vi "Compile Routines.vi"(8 "error in (no error)":errorcluster, 9 "Routines":T5[](array[typedef]) {"Stop Parameters"."Response"."Byte Order" items=["Little Endian", "Big Endian"]; "Stop Parameters"."Response"."Data Type" items=["Signed", "Unsigned", "IEEE Float"]; "Stop Parameters"."Cmd"."Byte Order" items=["Little Endian", "Big Endian"]; "Stop Parameters"."Cmd"."Data Type" items=["Signed", "Unsigned", "IEEE Float"]; "Request Parameters"."Response"."Byte Order" items=["Little Endian", "Big Endian"]; "Request Parameters"."Response"."Data Type" items=["Signed", "Unsigned", "IEEE Float"]; "Request Parameters"."Cmd"."Byte Order" items=["Little Endian", "Big Endian"]; "Request Parameters"."Cmd"."Data Type" items=["Signed", "Unsigned", "IEEE Float"]; "Start Parameters"."Response"."Byte Order" items=["Little Endian", "Big Endian"]; "Start Parameters"."Response"."Data Type" items=["Signed", "Unsigned", "IEEE Float"]; "Start Parameters"."Cmd"."Byte Order" items=["Little Endian", "Big Endian"]; "Start Parameters"."Cmd"."Data Type" items=["Signed", "Unsigned", "IEEE Float"]}, 10 "Routine Refs":T8[](array[typedef]) {"Stop"."Cmd Refs" format="%.0x"; "Stop"."Resp Refs" format="%.0x"; "Status"."Cmd Refs" format="%.0x"; "Status"."Resp Refs" format="%.0x"; "Start"."Cmd Refs" format="%.0x"; "Start"."Resp Refs" format="%.0x"}, 11 "Item Ref in":T10 format="%.0x") -> (0 "error out":errorcluster, 1 "Refs":T2 {"Stop.Resp" format="%.0x"; "Stop.Cmds"."Refs"."Data Reference" format="%.0x"; "Request.Resp" format="%.0x"; "Request.Cmds"."Refs"."Data Reference" format="%.0x"; "Start.Resp" format="%.0x"; "Start.Cmds"."Refs"."Data Reference" format="%.0x"}, 2 "Lookups":T1, 3 "Item Ref out":T10=18446744073709551615 format="%.0x")   [LabVIEW 2015, in "Diagnostics Addon System Explorer.lvlib"]
uses:
  Diagnostics Addon System Explorer.lvlib
  <vilib>/NI Veristand/Custom Device API/Custom Device Item Ref.ctl
  Types/Routine VS References.ctl
  Shared/Types/CmdResp Refs.ctl
  Shared/Types/Routine Paramaters.ctl
  Shared/Types/Command Response Signals.ctl
  Shared/Types/Signal Parameters.ctl
  Shared/Types/Compiled Routine Refs.ctl
  <vilib>/NI Veristand/Custom Device API/Block Data Reference.ctl
  <vilib>/NI Veristand/Custom Device API/Data Reference.ctl
  Shared/Types/Compiled Routine Lookups.ctl
  <vilib>/NI Veristand/Custom Device API/Data Access Type.ctl
  Shared/Types/Datatable Lookup Positions.ctl
  Shared/Diagnostics Addon Shared.lvlib
  <vilib>/NI Veristand/Custom Device API/Custom Device API.lvlib
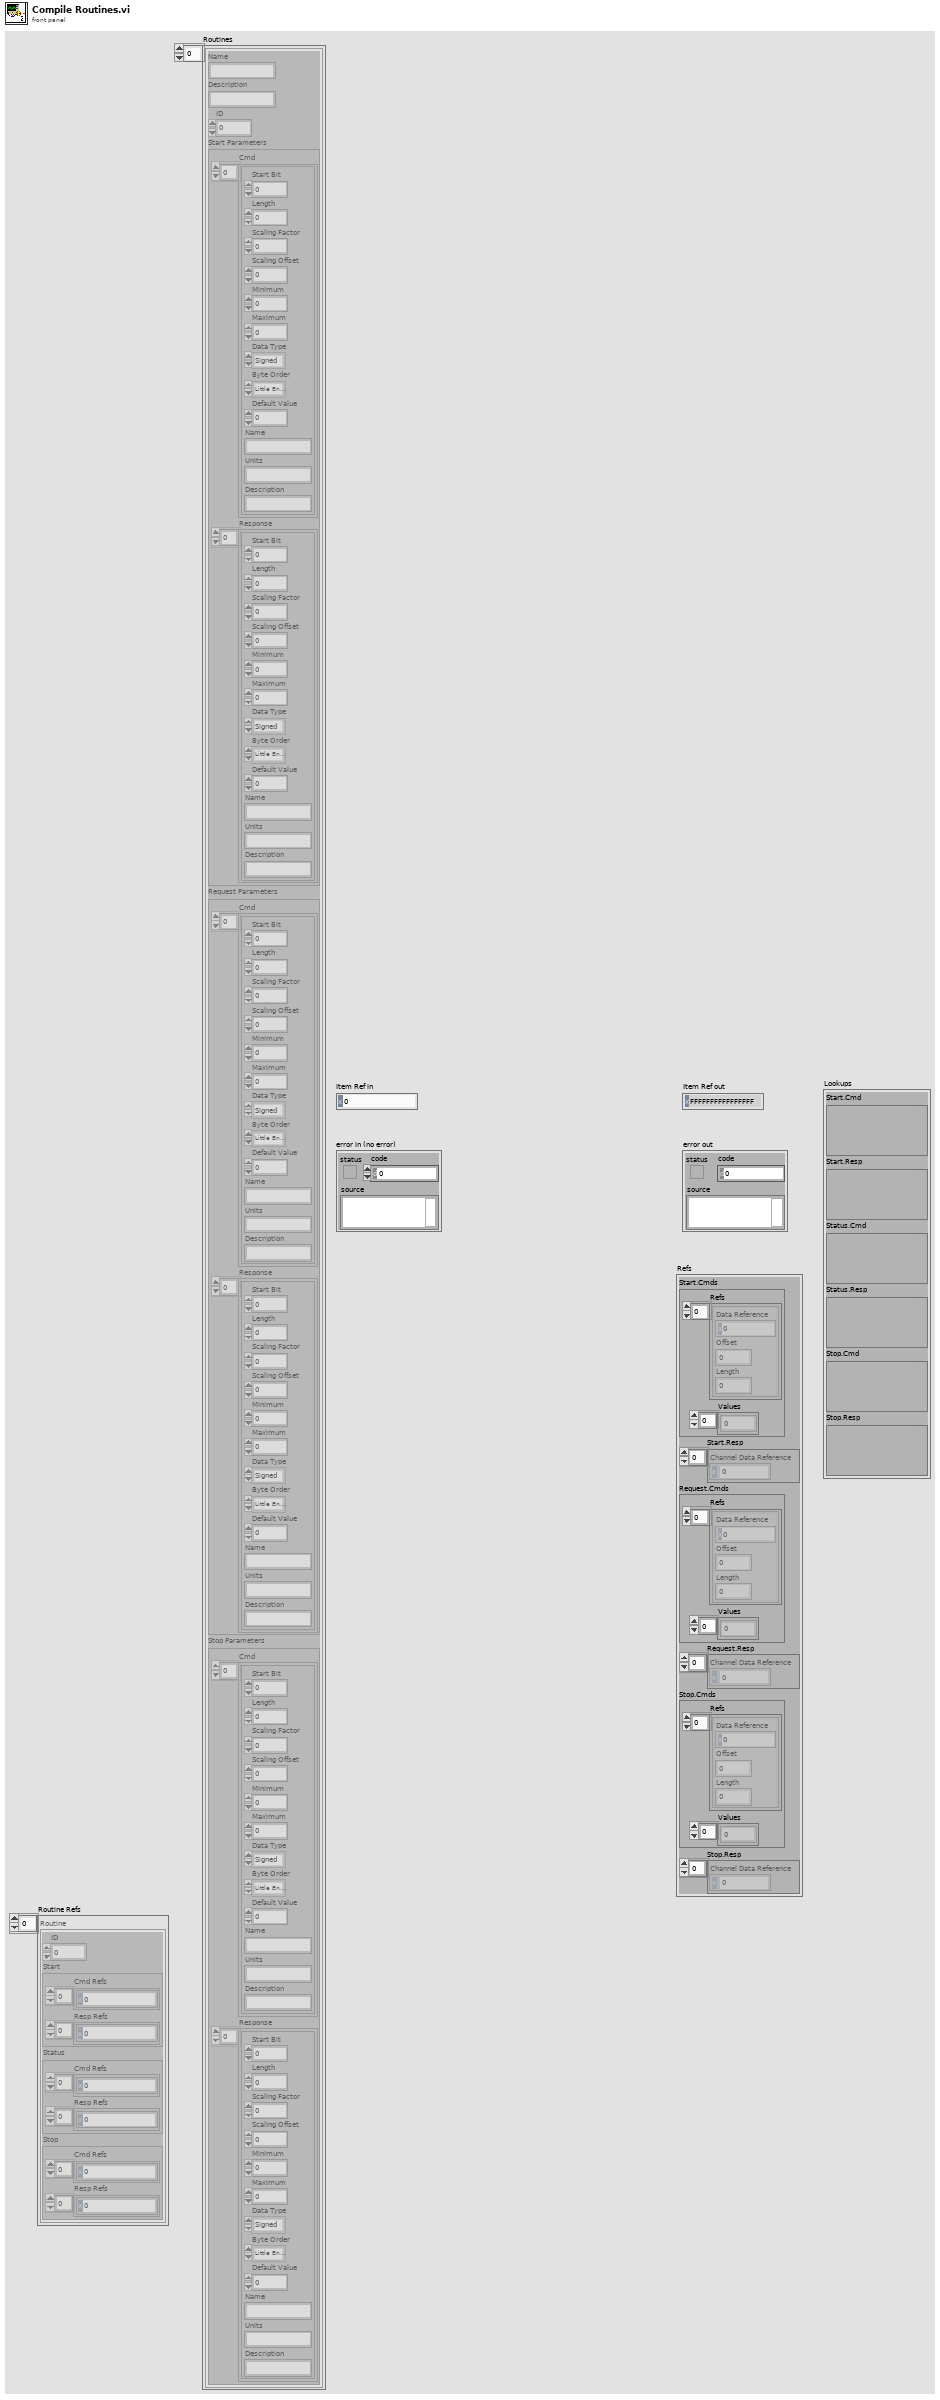
[diagram p1: front panel]
types:
  T1 = typedef "Diagnostics Addon Shared.lvlib/Compiled Routine Lookups.ctl" = cluster{"Start.Cmd":variant, "Start.Resp":variant, "Status.Cmd":variant, "Status.Resp":variant, "Stop.Cmd":variant, "Stop.Resp":variant}
  T2 = typedef "Diagnostics Addon Shared.lvlib/Compiled Routine Refs.ctl" = cluster{"Start.Cmds":cluster{"Refs":T3[], "Values":dbl[]}, "Start.Resp":T4[], "Request.Cmds":cluster{"Refs":T3[], "Values":dbl[]}, "Request.Resp":T4[], "Stop.Cmds":cluster{"Refs":T3[], "Values":dbl[]}, "Stop.Resp":T4[]}
  T3 = typedef "Custom Device API.lvlib/Block Data Reference.ctl" = cluster{"Data Reference":T4, "Offset":u64, "Length":u64}
  T4 = typedef "Custom Device API.lvlib/Data Reference.ctl" = i32
  T5 = typedef "Diagnostics Addon Shared.lvlib/Routine Paramaters.ctl" = cluster{"Name":string, "Description":string, "ID":u16, "Start Parameters":T6, "Request Parameters":T6, "Stop Parameters":T6}
  T6 = typedef "Diagnostics Addon Shared.lvlib/Command Response Signals.ctl" = cluster{"Cmd":T7[], "Response":T7[]}
  T7 = typedef "Diagnostics Addon Shared.lvlib/Signal Parameters.ctl" = cluster{"Start Bit":u8, "Length":u8, "Scaling Factor":dbl, "Scaling Offset":dbl, "Minimum":dbl, "Maximum":dbl, "Data Type":u32, "Byte Order":u32, "Default Value":dbl, "Name":string, "Units":string, "Description":string}
  T8 = typedef "Diagnostics Addon System Explorer.lvlib/Routine VS References.ctl" = cluster{"ID":u32, "Start":T9, "Status":T9, "Stop":T9}
  T9 = typedef "Diagnostics Addon Shared.lvlib/CmdResp Refs.ctl" = cluster{"Cmd Refs":T10[], "Resp Refs":T10[]}
  T10 = typedef "Custom Device API.lvlib/Custom Device Item Ref.ctl" = u64
  T11 = typedef "Custom Device API.lvlib/Data Access Type.ctl" = enum16{"Read", "Write"}
  T12 = typedef "Diagnostics Addon Shared.lvlib/Datatable Lookup Positions.ctl" = cluster{"Offset":i32, "Length":i32, "ByteLength":u16}
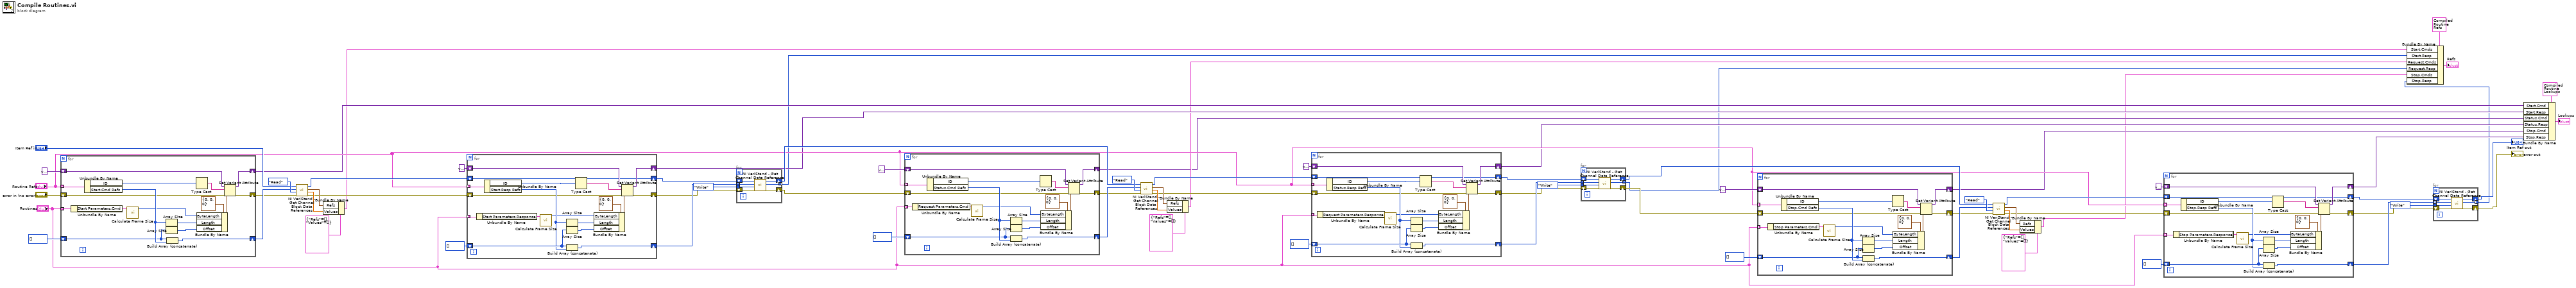
[diagram p0: block diagram]
diagram:
  n1 = for {
    tunnel: "Routine Refs" -> [w83] mode=indexing
    shift-right: [w84] -> w14
    shift-left: variant -> [w88]
    shift-right: [w86] -> w65
    shift-left: "error in (no error)" -> [w79]
    shift-right: [w82] -> w70
    shift-left: T10[] [] -> [w80]
    tunnel: "Routines" -> [w78] mode=indexing
    n2 = Unbundle By Name(w78) -> ("Start Parameters.Cmd"=w77:T7[])
    n3 = Unbundle By Name(w83) -> ("ID"=w75:u32, "Start.Cmd Refs"=w81:T10[])
    n4 = call "Calculate Frame Size.vi"("Parameters"=w77) -> ("Bytes"=w76:u16)  [unwired: 10 in]
    n5 = Array Size(array=w81) -> (size(s)=w91:i32)
    n6 = Array Size(array=w80) -> (size(s)=w87:i32)
    n7 = Build Array (concatenate)(w80, w81) -> (w82:T10[])
    n8 = Type Cast(x=w75) -> (*(type *) &x=w85:string)  [unwired: 1 in]
    n9 = Bundle By Name(cluster=T12 {"Offset"=0, "Length"=0, "ByteLength"=0}, "ByteLength"=w76, "Length"=w91, "Offset"=w87) -> (w89:T12)
    n10 = Set Variant Attribute(Variant=w88, name=w85, value=w89, error in=w79) -> (Variant out=w84:variant, error out=w86:errorcluster)  [unwired: 1 out]
  }
  n11 = call <vilib>:"NI VeriStand - Get Channel Block Data References.vi"("error in (no error)"=w65, "Access"=Data_Access_Type."Read", "Channel Refs"=w70, "Device Ref in"="Item Ref in") -> ("error out"=w58:errorcluster, "Values Array"=w66:dbl[], "Block Data Refs"=w67:T3[], "Device Ref out"=w57:T10)  [unwired: 4 in]
  n12 = Bundle By Name(cluster=cluster{"Refs":T3[], "Values":dbl[]} {"Refs"=[], "Values"=[]} ("Pairs"), "Refs"=w67, "Values"=w66) -> (w13:cluster{"Refs":T3[], "Values":dbl[]})
  n13 = for {
    tunnel: "Routine Refs" -> [w99] mode=indexing
    shift-right: [w108] -> w60
    shift-left: T10[] [] ("Signal Refs") -> [w109]
    shift-right: [w100] -> w12
    shift-left: variant -> [w104]
    shift-right: [w102] -> w59
    shift-left: w58 -> [w97]
    shift-right: [w96] -> w61
    shift-left: w57 -> [w96]
    tunnel: "Routines" -> [w95] mode=indexing
    n14 = Unbundle By Name(w95) -> ("Start Parameters.Response"=w94:T7[])
    n15 = Unbundle By Name(w99) -> ("ID"=w92:u32, "Start.Resp Refs"=w98:T10[])
    n16 = call "Calculate Frame Size.vi"("Parameters"=w94) -> ("Bytes"=w93:u16)  [unwired: 10 in]
    n17 = Array Size(array=w98) -> (size(s)=w107:i32)
    n18 = Array Size(array=w109) -> (size(s)=w103:i32)
    n19 = Build Array (concatenate)(w109, w98) -> (w108:T10[])
    n20 = Type Cast(x=w92) -> (*(type *) &x=w101:string)  [unwired: 1 in]
    n21 = Bundle By Name(cluster=T12 {"Offset"=0, "Length"=0, "ByteLength"=0}, "ByteLength"=w93, "Length"=w107, "Offset"=w103) -> (w105:T12)
    n22 = Set Variant Attribute(Variant=w104, name=w101, value=w105, error in=w97) -> (Variant out=w100:variant, error out=w102:errorcluster)  [unwired: 1 out]
  }
  n23 = for {
    tunnel: w60 -> [w112] mode=indexing
    tunnel: Data_Access_Type."Write" ("Access") -> [w111]
    shift-right: [w114] -> w26
    shift-left: w59 -> [w115]
    shift-right: [w116] -> w25
    shift-left: w61 -> [w113]
    tunnel: [w110] -> w11 mode=indexing
    n24 = call <vilib>:"NI VeriStand - Get Channel Data Reference.vi"("error in (no error)"=w115, "Access"=w111, "Channel Ref in"=w112, "Device Ref in"=w113) -> ("error out"=w114:errorcluster, "Channel Data Reference"=w110:T4, "Device Ref out"=w116:T10)  [unwired: 5 in]
  }
  n25 = for {
    tunnel: "Routine Refs" -> [w125] mode=indexing
    shift-right: [w126] -> w9
    shift-left: variant -> [w130]
    shift-right: [w128] -> w50
    shift-left: w26 -> [w121]
    shift-right: [w124] -> w54
    shift-left: T10[] [] -> [w122]
    tunnel: "Routines" -> [w120] mode=indexing
    n26 = Unbundle By Name(w120) -> ("Request Parameters.Cmd"=w119:T7[])
    n27 = Unbundle By Name(w125) -> ("ID"=w117:u32, "Status.Cmd Refs"=w123:T10[])
    n28 = call "Calculate Frame Size.vi"("Parameters"=w119) -> ("Bytes"=w118:u16)  [unwired: 10 in]
    n29 = Array Size(array=w123) -> (size(s)=w133:i32)
    n30 = Array Size(array=w122) -> (size(s)=w129:i32)
    n31 = Build Array (concatenate)(w122, w123) -> (w124:T10[])
    n32 = Type Cast(x=w117) -> (*(type *) &x=w127:string)  [unwired: 1 in]
    n33 = Bundle By Name(cluster=T12 {"Offset"=0, "Length"=0, "ByteLength"=0}, "ByteLength"=w118, "Length"=w133, "Offset"=w129) -> (w131:T12)
    n34 = Set Variant Attribute(Variant=w130, name=w127, value=w131, error in=w121) -> (Variant out=w126:variant, error out=w128:errorcluster)  [unwired: 1 out]
  }
  n35 = call <vilib>:"NI VeriStand - Get Channel Block Data References.vi"("error in (no error)"=w50, "Access"=Data_Access_Type."Read", "Channel Refs"=w54, "Device Ref in"=w25) -> ("error out"=w43:errorcluster, "Values Array"=w51:dbl[], "Block Data Refs"=w52:T3[], "Device Ref out"=w42:T10)  [unwired: 4 in]
  n36 = Bundle By Name(cluster=cluster{"Refs":T3[], "Values":dbl[]} {"Refs"=[], "Values"=[]} ("Pairs"), "Refs"=w52, "Values"=w51) -> (w10:cluster{"Refs":T3[], "Values":dbl[]})
  n37 = for {
    tunnel: "Routine Refs" -> [w141] mode=indexing
    shift-right: [w150] -> w45
    shift-left: T10[] [] ("Signal Refs") -> [w151]
    shift-right: [w142] -> w8
    shift-left: variant -> [w146]
    shift-right: [w144] -> w44
    shift-left: w43 -> [w139]
    shift-right: [w138] -> w46
    shift-left: w42 -> [w138]
    tunnel: "Routines" -> [w137] mode=indexing
    n38 = Unbundle By Name(w137) -> ("Request Parameters.Response"=w136:T7[])
    n39 = Unbundle By Name(w141) -> ("ID"=w134:u32, "Status.Resp Refs"=w140:T10[])
    n40 = call "Calculate Frame Size.vi"("Parameters"=w136) -> ("Bytes"=w135:u16)  [unwired: 10 in]
    n41 = Array Size(array=w140) -> (size(s)=w149:i32)
    n42 = Array Size(array=w151) -> (size(s)=w145:i32)
    n43 = Build Array (concatenate)(w151, w140) -> (w150:T10[])
    n44 = Type Cast(x=w134) -> (*(type *) &x=w143:string)  [unwired: 1 in]
    n45 = Bundle By Name(cluster=T12 {"Offset"=0, "Length"=0, "ByteLength"=0}, "ByteLength"=w135, "Length"=w149, "Offset"=w145) -> (w147:T12)
    n46 = Set Variant Attribute(Variant=w146, name=w143, value=w147, error in=w139) -> (Variant out=w142:variant, error out=w144:errorcluster)  [unwired: 1 out]
  }
  n47 = for {
    tunnel: w45 -> [w154] mode=indexing
    tunnel: Data_Access_Type."Write" ("Access") -> [w153]
    shift-right: [w156] -> w22
    shift-left: w44 -> [w157]
    shift-right: [w158] -> w21
    shift-left: w46 -> [w155]
    tunnel: [w152] -> w7 mode=indexing
    n48 = call <vilib>:"NI VeriStand - Get Channel Data Reference.vi"("error in (no error)"=w157, "Access"=w153, "Channel Ref in"=w154, "Device Ref in"=w155) -> ("error out"=w156:errorcluster, "Channel Data Reference"=w152:T4, "Device Ref out"=w158:T10)  [unwired: 5 in]
  }
  n49 = for {
    tunnel: "Routine Refs" -> [w167] mode=indexing
    shift-right: [w168] -> w6
    shift-left: variant -> [w172]
    shift-right: [w170] -> w35
    shift-left: w22 -> [w163]
    shift-right: [w166] -> w39
    shift-left: T10[] [] -> [w164]
    tunnel: "Routines" -> [w162] mode=indexing
    n50 = Unbundle By Name(w162) -> ("Stop Parameters.Cmd"=w161:T7[])
    n51 = Unbundle By Name(w167) -> ("ID"=w159:u32, "Stop.Cmd Refs"=w165:T10[])
    n52 = call "Calculate Frame Size.vi"("Parameters"=w161) -> ("Bytes"=w160:u16)  [unwired: 10 in]
    n53 = Array Size(array=w165) -> (size(s)=w175:i32)
    n54 = Array Size(array=w164) -> (size(s)=w171:i32)
    n55 = Build Array (concatenate)(w164, w165) -> (w166:T10[])
    n56 = Type Cast(x=w159) -> (*(type *) &x=w169:string)  [unwired: 1 in]
    n57 = Bundle By Name(cluster=T12 {"Offset"=0, "Length"=0, "ByteLength"=0}, "ByteLength"=w160, "Length"=w175, "Offset"=w171) -> (w173:T12)
    n58 = Set Variant Attribute(Variant=w172, name=w169, value=w173, error in=w163) -> (Variant out=w168:variant, error out=w170:errorcluster)  [unwired: 1 out]
  }
  n59 = call <vilib>:"NI VeriStand - Get Channel Block Data References.vi"("error in (no error)"=w35, "Access"=Data_Access_Type."Read", "Channel Refs"=w39, "Device Ref in"=w21) -> ("error out"=w28:errorcluster, "Values Array"=w36:dbl[], "Block Data Refs"=w37:T3[], "Device Ref out"=w27:T10)  [unwired: 4 in]
  n60 = Bundle By Name(cluster=cluster{"Refs":T3[], "Values":dbl[]} {"Refs"=[], "Values"=[]} ("Pairs"), "Refs"=w37, "Values"=w36) -> (w5:cluster{"Refs":T3[], "Values":dbl[]})
  n61 = for {
    tunnel: "Routine Refs" -> [w183] mode=indexing
    shift-right: [w192] -> w30
    shift-left: T10[] [] ("Signal Refs") -> [w193]
    shift-right: [w184] -> w4
    shift-left: variant -> [w188]
    shift-right: [w186] -> w29
    shift-left: w28 -> [w181]
    shift-right: [w180] -> w31
    shift-left: w27 -> [w180]
    tunnel: "Routines" -> [w179] mode=indexing
    n62 = Unbundle By Name(w179) -> ("Stop Parameters.Response"=w178:T7[])
    n63 = Unbundle By Name(w183) -> ("ID"=w176:u32, "Stop.Resp Refs"=w182:T10[])
    n64 = call "Calculate Frame Size.vi"("Parameters"=w178) -> ("Bytes"=w177:u16)  [unwired: 10 in]
    n65 = Array Size(array=w182) -> (size(s)=w191:i32)
    n66 = Array Size(array=w193) -> (size(s)=w187:i32)
    n67 = Build Array (concatenate)(w193, w182) -> (w192:T10[])
    n68 = Type Cast(x=w176) -> (*(type *) &x=w185:string)  [unwired: 1 in]
    n69 = Bundle By Name(cluster=T12 {"Offset"=0, "Length"=0, "ByteLength"=0}, "ByteLength"=w177, "Length"=w191, "Offset"=w187) -> (w189:T12)
    n70 = Set Variant Attribute(Variant=w188, name=w185, value=w189, error in=w181) -> (Variant out=w184:variant, error out=w186:errorcluster)  [unwired: 1 out]
  }
  n71 = for {
    tunnel: w30 -> [w196] mode=indexing
    tunnel: Data_Access_Type."Write" ("Access") -> [w195]
    shift-right: [w198] -> w18
    shift-left: w29 -> [w199]
    shift-right: [w200] -> w17
    shift-left: w31 -> [w197]
    tunnel: [w194] -> w3 mode=indexing
    n72 = call <vilib>:"NI VeriStand - Get Channel Data Reference.vi"("error in (no error)"=w199, "Access"=w195, "Channel Ref in"=w196, "Device Ref in"=w197) -> ("error out"=w198:errorcluster, "Channel Data Reference"=w194:T4, "Device Ref out"=w200:T10)  [unwired: 5 in]
  }
  "error out" <- w18
  "Item Ref out" <- w17
  n73 = Bundle By Name(cluster=T2 {"Start.Cmds"={"Refs"=[], "Values"=[]}, "Start.Resp"=[], "Request.Cmds"={"Refs"=[], "Values"=[]}, "Request.Resp"=[], "Stop.Cmds"={"Refs"=[], "Values"=[]}, "Stop.Resp"=[]} ("Routine Refs"), "Start.Cmds"=w13, "Start.Resp"=w11, "Request.Cmds"=w10, "Request.Resp"=w7, "Stop.Cmds"=w5, "Stop.Resp"=w3) -> (→"Refs":T2)
  n74 = Bundle By Name(cluster=T1 {"Start.Cmd"=variant, "Start.Resp"=variant, "Status.Cmd"=variant, "Status.Resp"=variant, "Stop.Cmd"=variant, "Stop.Resp"=variant} ("Routine Lookups"), "Start.Cmd"=w14, "Start.Resp"=w12, "Status.Cmd"=w9, "Status.Resp"=w8, "Stop.Cmd"=w6, "Stop.Resp"=w4) -> (→"Lookups":T1)
